vi "Case Key Structure1111.vi"() -> ()   [LabVIEW 2012]
panel:
  out "Case Key":i32
  out "Case 5":i32
  out "Case 4":i32
  out "Case 3":i32
  out "Numeric 4":i32
  out "Numeric 3":i32
  out "Numeric 2":i32
  out "Numeric":i32
  out "Case 2":i32
  in  "TF in Air":i32
  out "Control Signal1":i32
  in  "Approach Minimum":i32
  in  "Approach Setpoint":i32
  in  "Fast Approach Offset":i32
  in  "Control Signal":i32
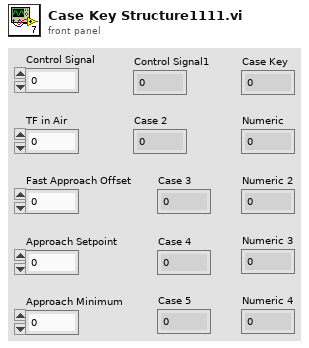
[diagram p1: front panel]
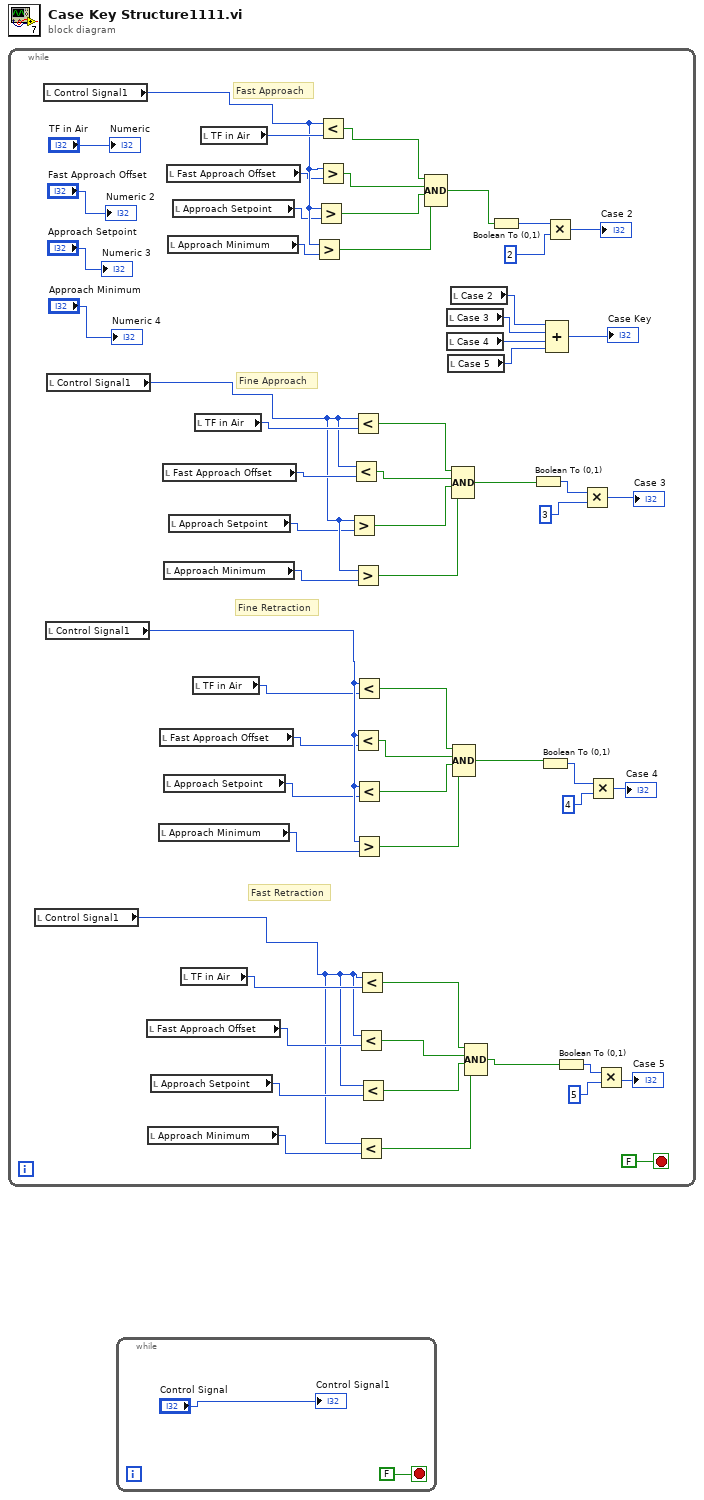
[diagram p0: block diagram]
diagram:
  n1 = while {
    stop <- FALSE stop-if-true
    # "Fast Retraction"
    # "Fine Retraction"
    # "Fine Approach"
    # "Fast Approach"
    n2 = local read "Control Signal1"() -> (w19:i32)
    n3 = local read "Control Signal1"() -> (w59:i32)
    n4 = local read "Control Signal1"() -> (w31:i32)
    n5 = local read "Control Signal1"() -> (w42:i32)
    n6 = local read "Fast Approach Offset"() -> (w21:i32)
    n7 = local read "Approach Minimum"() -> (w18:i32)
    n8 = local read "Approach Setpoint"() -> (w20:i32)
    n9 = local read "Approach Minimum"() -> (w27:i32)
    n10 = local read "Fast Approach Offset"() -> (w29:i32)
    n11 = local read "Fast Approach Offset"() -> (w43:i32)
    n12 = local read "Approach Minimum"() -> (w40:i32)
    n13 = local read "Approach Setpoint"() -> (w28:i32)
    n14 = local read "Fast Approach Offset"() -> (w58:i32)
    n15 = local read "Approach Minimum"() -> (w56:i32)
    n16 = local read "Approach Setpoint"() -> (w41:i32)
    n17 = local read "Approach Setpoint"() -> (w57:i32)
    n18 = local read "TF in Air"() -> (w22:i32)
    n19 = local read "TF in Air"() -> (w30:i32)
    n20 = local read "TF in Air"() -> (w44:i32)
    n21 = local read "TF in Air"() -> (w61:i32)
    n22 = Greater?(x=w59, y=w56) -> (0:w53:bool)
    n23 = Greater?(x=w59, y=w57) -> (0:w54:bool)
    n24 = Less?(x=w59, y=w61) -> (x < y?=w60:bool)
    n25 = Greater?(x=w59, y=w58) -> (0:w55:bool)
    n26 = Greater?(x=w42, y=w41) -> (0:w37:bool)
    n27 = Less?(x=w42, y=w43) -> (x < y?=w38:bool)
    n28 = Less?(x=w42, y=w44) -> (x < y?=w39:bool)
    n29 = Greater?(x=w42, y=w40) -> (0:w36:bool)
    n30 = Less?(x=w31, y=w29) -> (x < y?=w25:bool)
    n31 = Less?(x=w31, y=w30) -> (x < y?=w26:bool)
    n32 = Less?(x=w31, y=w28) -> (x < y?=w24:bool)
    n33 = Greater?(x=w31, y=w27) -> (0:w23:bool)
    n34 = Less?(x=w19, y=w21) -> (x < y?=w16:bool)
    n35 = Less?(x=w19, y=w18) -> (x < y?=w14:bool)
    n36 = Less?(x=w19, y=w22) -> (x < y?=w17:bool)
    n37 = Less?(x=w19, y=w20) -> (x < y?=w15:bool)
    n38 = Compound Arithmetic op=AND(w60, w55, w54, w53) -> (w52:bool)
    n39 = local read "Case 3"() -> (w4:i32)
    n40 = local read "Case 4"() -> (w3:i32)
    n41 = local read "Case 5"() -> (w2:i32)
    n42 = local read "Case 2"() -> (w5:i32)
    n43 = Compound Arithmetic op=AND(w39, w38, w37, w36) -> (w35:bool)
    n44 = Compound Arithmetic op=AND(w26, w25, w24, w23) -> (w12:bool)
    n45 = Compound Arithmetic op=AND(w17, w16, w15, w14) -> (w13:bool)
    n46 = Boolean To (0,1)(Boolean=w52) -> (0, 1=w50:i16)
    n47 = Boolean To (0,1)(Boolean=w35) -> (0, 1=w34:i16)
    n48 = Boolean To (0,1)(Boolean=w12) -> (0, 1=w10:i16)
    n49 = Multiply(x=w50, y=2) -> (x*y=→"Case 2":i32)
    n50 = Compound Arithmetic op=ADD(w5, w4, w3, w2) -> (→"Case Key":i32)
    n51 = Boolean To (0,1)(Boolean=w13) -> (0, 1=w11:i16)
    n52 = Multiply(x=w34, y=3) -> (x*y=→"Case 3":i32)
    n53 = Multiply(x=w10, y=4) -> (x*y=→"Case 4":i32)
    n54 = Multiply(x=w11, y=5) -> (x*y=→"Case 5":i32)
    "Numeric" <- "TF in Air"
    "Numeric 2" <- "Fast Approach Offset"
    "Numeric 3" <- "Approach Setpoint"
    "Numeric 4" <- "Approach Minimum"
  }
  n55 = while {
    stop <- FALSE stop-if-true
    "Control Signal1" <- "Control Signal"
  }
